vi "SEQPoolFGV.vi"(9 "Action":T1(ring), 10 "Index":i8, 11 "SEQ in":refnum<class "Sequence.lvclass">) -> (1 "Pool out":refnum<class "Sequence.lvclass">[](array[class]), 2 "Size":i8, 3 "SEQ out":refnum<class "Sequence.lvclass">)   [LabVIEW 2012, in "StimulCtrls.lvlib"]
uses:
  StimulCtrls.lvlib
  Sequence.lvclass
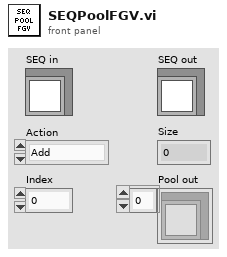
[diagram p1: front panel]
types:
  T1 = enum16{"Add", "New", "Del", "Update", "Get", "Initial", "GetSize"}
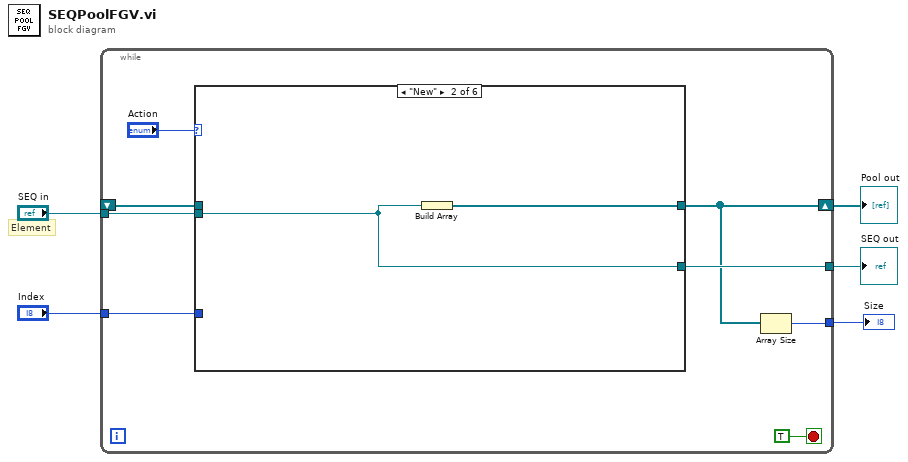
[diagram p0: block diagram]
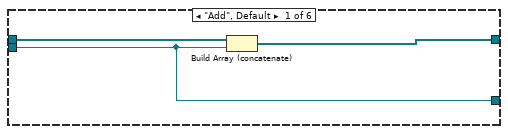
[diagram p2: hidden frame]
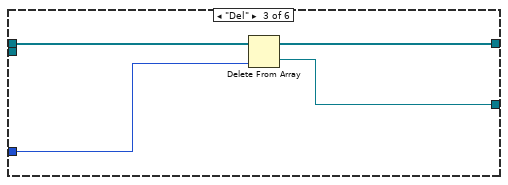
[diagram p3: hidden frame]
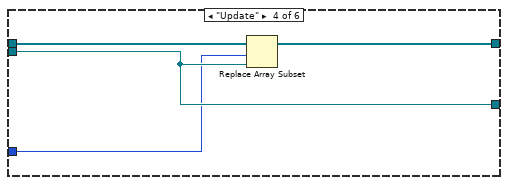
[diagram p4: hidden frame]
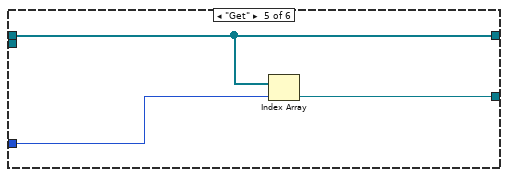
[diagram p5: hidden frame]
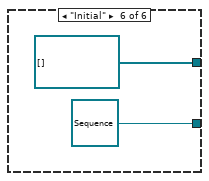
[diagram p6: hidden frame]
diagram:
  # "Element"
  n1 = while {
    tunnel: "SEQ in" -> [w11]
    shift-right: [w7] -> w2
    shift-left: _ -> [w10]
    tunnel: [w9] -> w4
    tunnel: [w8] -> w3
    tunnel: "Index" -> [w6]
    stop <- TRUE stop-if-true
    n2 = case shown="\"New\"" "Action" {
      tunnel: w11 -> [w14 w17 _ w24 _ _]
      tunnel: w10 -> [w16 _ w22 w26 w29 _]
      tunnel: [w15 w18 w20 w25 w29 refnum<class "Sequence.lvclass">[] []] -> w7
      tunnel: w6 -> [_ _ w21 w23 w28 _]
      tunnel: [w14 w17 w19 w24 w27 refnum<class "Sequence.lvclass"> refnum ("Sequence.lvclass")] -> w9
      frame "Add", Default {
        n3 = Build Array (concatenate)(w16, w14) -> (w15:refnum<class "Sequence.lvclass">[])
      }
      frame "New" {
        n4 = Build Array(w17) -> (w18:refnum<class "Sequence.lvclass">[])
      }
      frame "Del" {
        n5 = Delete From Array(array=w22, index=w21) -> (deleted portion=w19:refnum<class "Sequence.lvclass">, array with subset deleted=w20:refnum<class "Sequence.lvclass">[])  [unwired: 1 in]
      }
      frame "Update" {
        n6 = Replace Array Subset(array=w26, new element=w24, index=w23) -> (w25:refnum<class "Sequence.lvclass">[])
      }
      frame "Get" {
        n7 = Index Array(array=w29, index=w28) -> (element=w27:refnum<class "Sequence.lvclass">)
      }
      frame "Initial" {
      }
    }
    n8 = Array Size(array=w7) -> (size(s)=w8:i32)
  }
  "SEQ out" <- w4
  "Size" <- w3
  "Pool out" <- w2
